vi "niRFUtil LCAPI Copy WFM (3 SGL).vi"(0 "Source0 WFM (SGL)":T1 {"y" min=0 max=127 format="%.2f"; "dx" format="%^.2e"; "x0" format="%^.2e"}, 5 "Source1 WFM (SGL)":T1 {"y" min=0 max=127 format="%.2f"; "dx" format="%^.2e"; "x0" format="%^.2e"}, 7 "Source2 WFM (SGL)":T1 {"y" min=0 max=127 format="%.2f"; "dx" format="%^.2e"; "x0" format="%^.2e"}, 11 "error in (no error)":errorcluster, 12 "Data Copy Descriptor":u64) -> (4 "Source0 Out":T1 {"y" min=0 max=127 format="%.2f"; "dx" format="%^.2e"; "x0" format="%^.2e"}, 6 "Source1 Out":T1 {"y" min=0 max=127 format="%.2f"; "dx" format="%^.2e"; "x0" format="%^.2e"}, 8 "Source2 Out":T1 {"y" min=0 max=127 format="%.2f"; "dx" format="%^.2e"; "x0" format="%^.2e"}, 15 "error out":errorcluster)   [LabVIEW 2015, in "niRFUtil.lvlib"]
uses:
  niRFUtil.lvlib
  Includes/niRFUtil INC Real Waveform.ctl
  Includes/niRFUtil INC Real Array.ctl
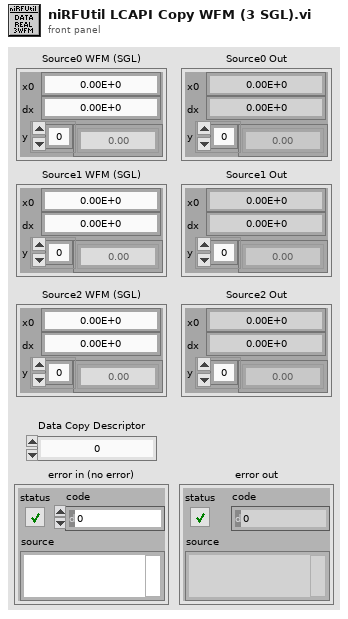
[diagram p1: front panel]
types:
  T1 = typedef "niRFUtil.lvlib/niRFUtil INC Real Waveform.ctl" = cluster{"x0":dbl, "dx":dbl, "y":T2}
  T2 = typedef "niRFUtil.lvlib/niRFUtil INC Real Array.ctl" = sgl[]
  T3 = cluster{"status":bool, "return type":i32, "errorString":string}
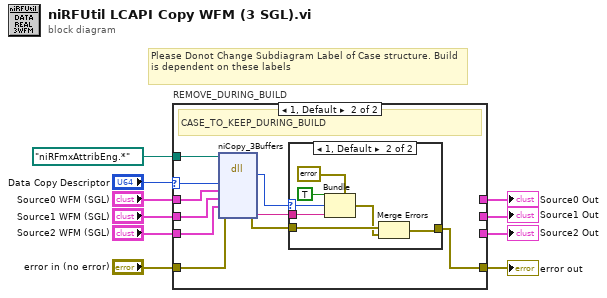
[diagram p0: block diagram]
diagram:
  # "Please Donot Change Subdiagram Label of Case structure. Build is dependent on these labels"
  n1 = case "REMOVE_DURING_BUILD" shown="1, Default" "Data Copy Descriptor" {
    selector: "Data Copy Descriptor" -> [_ w17]
    tunnel: "Source0 WFM (SGL)" -> [w14 w24]
    tunnel: "error in (no error)" -> [w11 w23]
    tunnel: "Source1 WFM (SGL)" -> [w13 w22]
    tunnel: "Source2 WFM (SGL)" -> [w12 w21]
    tunnel: [w14 _] -> w5
    tunnel: [w13 _] -> w4
    tunnel: [w12 _] -> w3
    tunnel: [w11 w16] -> w2
    tunnel: path "niRFmxAttribEng.*" ("path in") -> [_ w15]
    frame 0 {
      # "Development"
    }
    frame 1, Default {
      # "CASE_TO_KEEP_DURING_BUILD"
      n2 = dll-call lib="niRFmxAttribEng.*" fn="niCopy_3Buffers"(path in=w15, error in=w23, "dataCopyDescriptor"=w17, "source0"=w24, "source1"=w22, "source2"=w21) -> (error out=w18:errorcluster, "return type"=w19:i32, "errorString"=w20:string)  [unwired: 6 in, 1 out]
      n3 = case shown="1, Default" w19 {
        selector: w19 -> [_ w29]
        tunnel: w20 -> [_ w30]
        tunnel: w18 -> [w25 w32]
        tunnel: [w25 w31] -> w16
        frame 0 {
        }
        frame 1, Default {
          n4 = Bundle(cluster=T3 {"status"=FALSE, "return type"=0, "errorString"=""}, "status"=TRUE, "return type"=w29, "errorString"=w30) -> (w26:T3)
          n5 = Merge Errors(w32, w26) -> (w31:errorcluster)
        }
      }
    }
  }
  "error out" <- w2
  "Source0 Out" <- w5
  "Source1 Out" <- w4
  "Source2 Out" <- w3
